vi "lecture2-Calculating Slope.vi"(8 "X1":dbl, 9 "Y2":dbl, 10 "Y1":dbl, 11 "X2":dbl) -> (3 "Slope (m)":dbl)   [LabVIEW 2014]
doc: "i don't care about this shit."
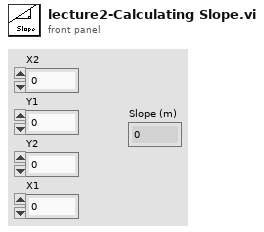
[diagram p1: front panel]
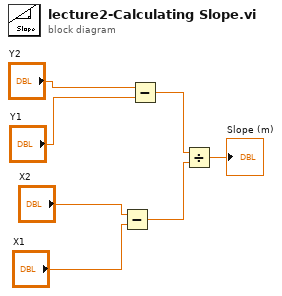
[diagram p0: block diagram]
diagram:
  n1 = Subtract(x="X2", y="X1") -> (x-y=w3:dbl)
  n2 = Subtract(x="Y2", y="Y1") -> (x-y=w2:dbl)
  n3 = Divide(x=w2, y=w3) -> (x/y=→"Slope (m)":dbl)
